vi "RedistributeArmPathPoints.vi"(0 "Angles":dbl[](array[numeric]), 1 "Path Length (in)":dbl, 2 "Desired Point Spacing (in)":dbl, 4 "Radii":dbl[](array[numeric]), 5 "IndexedPathLength":dbl[](array[numeric])) -> (3 "Angles Out":dbl[](array[numeric]), 7 "Radii Out":dbl[](array[numeric]))   [LabVIEW 2017]
uses:
  ArgosLib/ArgosLib.lvlib
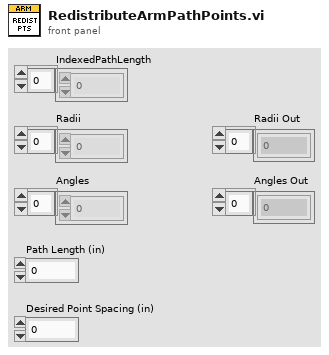
[diagram p1: front panel]
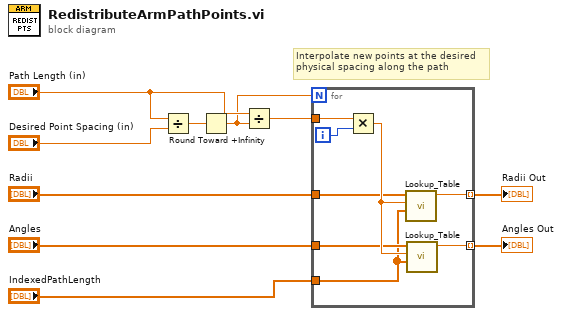
[diagram p0: block diagram]
diagram:
  # "Interpolate new points at the desired\nphysical spacing along the path"
  n1 = Divide(x="Path Length (in)", y="Desired Point Spacing (in)") -> (x/y=w9:dbl)
  n2 = Round Toward +Infinity(x=w9) -> (ceil(x): smallest int >= x=w3:dbl)
  n3 = Divide(x="Path Length (in)", y=w3) -> (x/y=w7:dbl)
  n4 = for {
    N: w3 -> [_]
    tunnel: w7 -> [w17]
    tunnel: "Radii" -> [w15]
    tunnel: "Angles" -> [w14]
    tunnel: "IndexedPathLength" -> [w13]
    tunnel: [w12] -> w2 mode=indexing
    tunnel: [w11] -> w1 mode=indexing
    i -> [w18]
    n5 = Multiply(x=w17, y=w18) -> (x*y=w16:dbl)
    n6 = call "Lookup_Table.vi"("Y_Array"=w15, "x_in"=w16, "X_Array"=w13) -> ("y_out"=w11:dbl)  [unwired: 6 in]
    n7 = call "Lookup_Table.vi"("Y_Array"=w14, "x_in"=w16, "X_Array"=w13) -> ("y_out"=w12:dbl)  [unwired: 6 in]
  }
  "Radii Out" <- w1
  "Angles Out" <- w2
